vi "Vent.vi"(8 "error in (no error)":errorcluster, 9 "Pressure threshold":dbl=0.01, 10 "Max vent time (s)":u32=10, 11 "Pressure Control in":refnum<class "Pressure Control.lvclass">) -> (0 "error out":errorcluster, 3 "Pressure Control out":refnum<class "Pressure Control.lvclass">)   [LabVIEW 2011, in "Pressure Control.lvclass"]
doc: "Vents the pressure chamber by opening up the \"Pressure down\" valve, until the pressure has dropped below the threshold value, or until \"Max vent time\" has passed."
uses:
  Pressure Control.lvclass
  Pressure Control.lvclass/Pressure Control.ctl
  TTL/TTL.lvclass
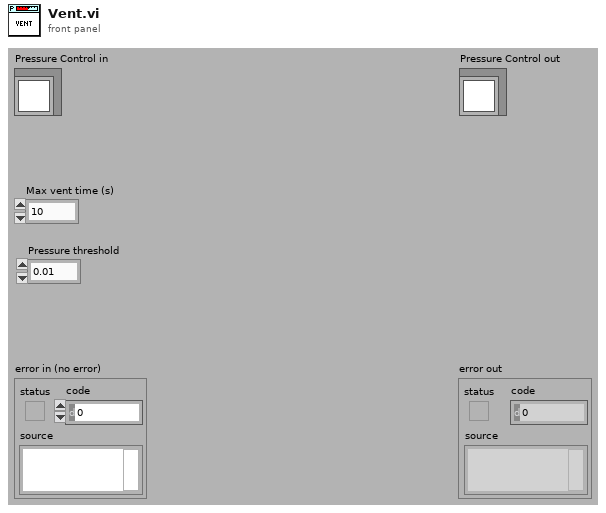
[diagram p1: front panel]
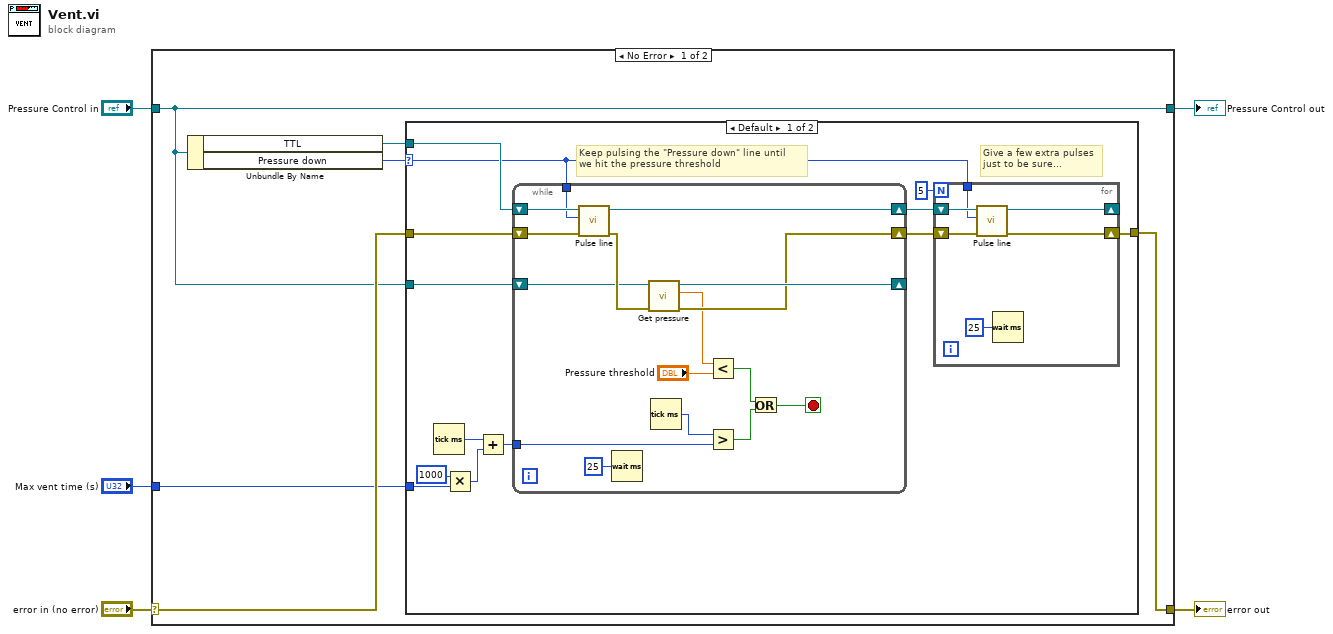
[diagram p0: block diagram]
diagram:
  n1 = case shown="No Error" "error in (no error)" {
    selector: "error in (no error)" -> [w9 w49]
    tunnel: [w8 w49] -> w4
    tunnel: [w6 w48] -> w2
    tunnel: "Pressure Control in" -> [w6 w48]
    tunnel: "Max vent time (s)" -> [w7 _]
    frame No Error {
      n2 = Unbundle By Name(w6) -> ("TTL"=w10:refnum<class "TTL.lvclass">, "Pressure down"=w11:i32)
      n3 = case shown="Default" w11 {
        selector: w11 -> [w12 _]
        tunnel: w10 -> [w18 _]
        tunnel: w9 -> [w17 w47]
        tunnel: [w14 w47] -> w8
        tunnel: w7 -> [w23 _]
        tunnel: w6 -> [w19 _]
        frame Default {
          # "Give a few extra pulses\njust to be sure..."
          # "Keep pulsing the \"Pressure down\" line until\nwe hit the pressure threshold"
          n4 = Tick Count (ms)() -> (millisecond timer value=w24:u32)
          n5 = Multiply(x=u32 1000, y=w23) -> (x*y=w21:u32)
          n6 = Add(x=w24, y=w21) -> (x+y=w20:u32)
          n7 = while {
            tunnel: w20 -> [w39]
            shift-right: [w43] -> _
            shift-left: w19 -> [w44]
            shift-right: [w42] -> w15
            shift-left: w17 -> [w33]
            shift-right: [w31] -> w16
            shift-left: w18 -> [w34]
            tunnel: w12 -> [w32]
            stop <- w35 stop-if-true
            n8 = call "Pulse line.vi"("error in (no error)"=w33, "Line number"=w32, "TTL in"=w34) -> ("error out"=w46:errorcluster, "TTL out"=w31:refnum<class "TTL.lvclass">)  [unwired: 7 in]
            n9 = Wait (ms)(milliseconds to wait=u32 25) -> ()  [unwired: 1 out]
            n10 = call "Get pressure.vi"("error in (no error)"=w46, "Pressure Control in"=w44) -> ("error out"=w42:errorcluster, "Pressure"=w41:dbl, "Pressure Control out"=w43:refnum<class "Pressure Control.lvclass">)  [unwired: 6 in, 1 out]
            n11 = Tick Count (ms)() -> (millisecond timer value=w38:u32)
            n12 = Less?(x=w41, y="Pressure threshold") -> (x < y?=w37:bool)
            n13 = Greater?(x=w38, y=w39) -> (0:w36:bool)
            n14 = Or(x=w37, y=w36) -> (x .or. y?=w35:bool)
          }
          n15 = for {
            N: 5 -> [_]
            shift-right: [w29] -> _
            shift-left: w16 -> [w30]
            shift-right: [w27] -> w14
            shift-left: w15 -> [w28]
            tunnel: w12 -> [w25]
            n16 = call "Pulse line.vi"("error in (no error)"=w28, "Line number"=w25, "TTL in"=w30) -> ("error out"=w27:errorcluster, "TTL out"=w29:refnum<class "TTL.lvclass">)  [unwired: 7 in]
            n17 = Wait (ms)(milliseconds to wait=u32 25) -> ()  [unwired: 1 out]
          }
        }
        frame -1 {
          # "No \"down\" line was defined\nin the hardware config"
        }
      }
    }
    frame Error {
    }
  }
  "error out" <- w4
  "Pressure Control out" <- w2
